vi "4town.vi"() -> ()   [LabVIEW 2021]
panel:
  out "XY Graph":cluster{i32[], dbl[]}[](graph)
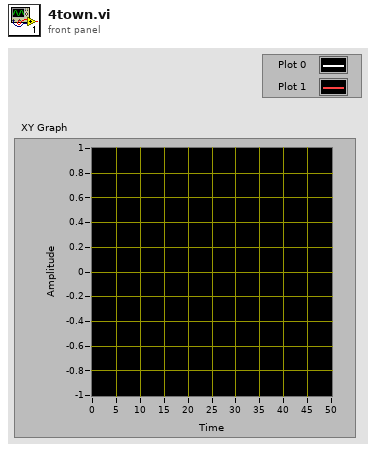
[diagram p1: front panel]
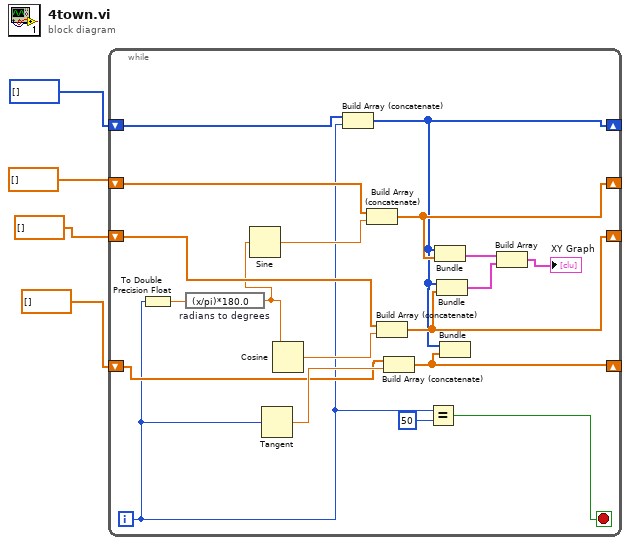
[diagram p0: block diagram]
diagram:
  n1 = while {
    shift-right: [w7] -> _
    shift-left: i32[] [] -> [w23]
    shift-right: [w19] -> _
    shift-left: dbl[] [] -> [w22]
    shift-right: [w11] -> _
    shift-left: dbl[] [] -> [w15]
    shift-right: [w6] -> _
    shift-left: dbl[] [] -> [w12]
    i -> [w5]
    stop <- w21 stop-if-true
    n2 = To Double Precision Float(number=w5) -> (double precision float=w18:dbl)
    n3 = expression code="(x/pi)*180.0" "radians to degrees"(w18) -> (w14:dbl)
    n4 = Sine(x=w14) -> (sin(x)=w17:dbl)
    n5 = Tangent(1:w5) -> (0:w13:dbl)
    n6 = Cosine(x=w14) -> (cos(x)=w16:dbl)
    n7 = Build Array (concatenate)(w23, w5) -> (w7:i32[])
    n8 = Build Array (concatenate)(w22, w17) -> (w19:dbl[])
    n9 = Build Array (concatenate)(w15, w16) -> (w11:dbl[])
    n10 = Build Array (concatenate)(w12, w13) -> (w6:dbl[])
    n11 = Equal?(x=w5, y=50) -> (x = y?=w21:bool)
    n12 = Bundle(w7, w19) -> (w10:cluster{i32[], dbl[]})  [unwired: 1 in]
    n13 = Bundle(w7, w11) -> (w9:cluster{i32[], dbl[]})  [unwired: 1 in]
    n14 = Bundle(w7, w6) -> ()  [unwired: 1 in, 1 out]
    n15 = Build Array(w10, w9) -> (→"XY Graph":cluster{i32[], dbl[]}[])
  }
